vi "SWERVE_SIM_MODULE_READ_ENCODERS.vi"(10 "FPGA_Time_Seconds":dbl=-1.0, 11 "Swerve Module TypDef":T1) -> (2 "Swerve Distance_Radians":dbl, 3 "Wheel Distance_Meters":dbl)   [LabVIEW 2019]
uses:
  <vilib>/Rock Robotics/WPI/ThirdParty/JAS_Junk/TrajLib/Trajectory_Library.lvlib
  <vilib>/Rock Robotics/SystemInterfaces/Encoder/FPGA_EncoderIdx.ctl
  <vilib>/Rock Robotics/WPI/Encoder/WPI_EncoderType.ctl
  <vilib>/Rock Robotics/SystemInterfaces/Counter/FPGA_CounterCtrSystemIndex.ctl
  <vilib>/Rock Robotics/WPI/Encoder/WPI_EncoderDevRef.ctl
  <vilib>/Rock Robotics/SystemInterfaces/DIO/FPGA_DIOPWMChannel.ctl
  <vilib>/Rock Robotics/WPI/PWM/WPI_PWMDeadband.ctl
  <vilib>/Rock Robotics/WPI/MotorControl/WPI_MotorControlType.ctl
  <vilib>/Rock Robotics/SystemInterfaces/DIO/FPGA_DIOChannel.ctl
  <vilib>/Rock Robotics/WPI/MotorControl/WPI_MotorControlDeviceRef.ctl
  Swerve_Drive_System/SWERVE_DRIVE_MODULE_TYPDEF.ctl
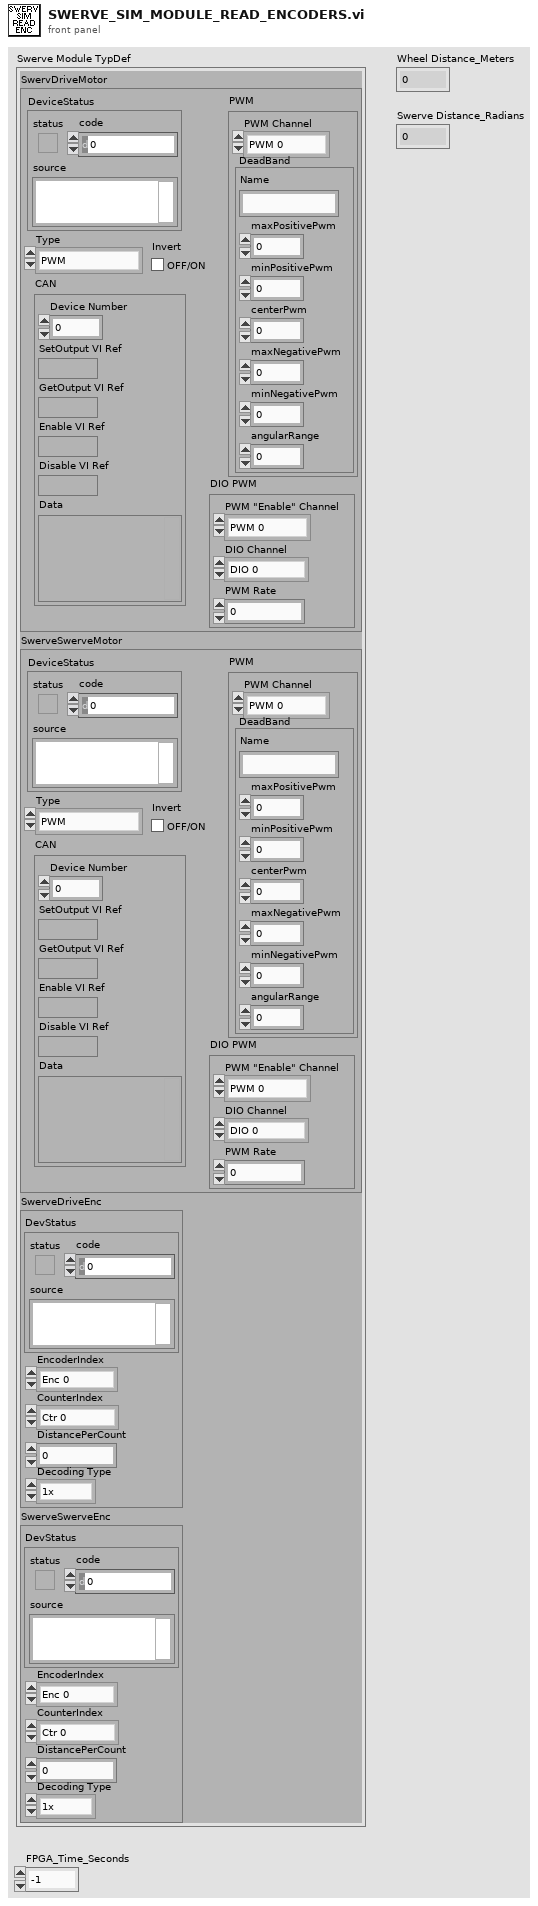
[diagram p1: front panel]
types:
  T1 = typedef "SWERVE_DRIVE_MODULE_TYPDEF.ctl" = cluster{"SwervDriveMotor":T2, "SwerveSwerveMotor":T2, "SwerveDriveEnc":T7, "SwerveSwerveEnc":T7}
  T2 = typedef "WPI_MotorControlDeviceRef.ctl" = cluster{"DeviceStatus":errorcluster, "Type":T3, "PWM":cluster{"PWM Channel":T4, "DeadBand":T5}, "CAN":cluster{"Device Number":u8, "SetOutput VI Ref":variant, "GetOutput VI Ref":variant, "Enable VI Ref":variant, "Disable VI Ref":variant, "Data":variant}, "Invert":bool, "DIO PWM":cluster{"PWM \"Enable\" Channel":T4, "DIOChannel":T6, "PWM Rate":dbl}}
  T3 = typedef "WPI_MotorControlType.ctl" = enum16{"PWM", "CAN", "DIO PWM"}
  T4 = typedef "FPGA_DIOPWMChannel.ctl" = enum8{"PWM 0", "PWM 1", "PWM 2", "PWM 3", "PWM 4", "PWM 5", "PWM 6", "PWM 7", "PWM 8", "PWM 9", "PWM MXP 0", "PWM MXP 1", "PWM MXP 2", "PWM MXP 3", "PWM MXP 4", "PWM MXP 5", "PWM MXP 6", "PWM MXP 7", "PWM MXP 8", "PWM MXP 9", "Invalid"}
  T5 = typedef "WPI_PWMDeadband.ctl" = cluster{"Name":string, "maxPositivePwm":i32, "minPositivePwm":i32, "centerPwm":i32, "maxNegativePwm":i32, "minNegativePwm":i32, "angularRange":u16}
  T6 = typedef "FPGA_DIOChannel.ctl" = enum8{"DIO 0", "DIO 1", "DIO 2", "DIO 3", "DIO 4", "DIO 5", "DIO 6", "DIO 7", "DIO 8", "DIO 9", "DIO MXP 0", "DIO MXP 1", "DIO MXP 2", "DIO MXP 3", "DIO MXP 4", "DIO MXP 5", "DIO MXP 6", "DIO MXP 7", "DIO MXP 8", "DIO MXP 9", "DIO MXP 10", "DIO MXP 11", "DIO MXP 12", "DIO MXP 13", "DIO MXP 14", "DIO MXP 15", "SPI Port CS1", "SPI Port CS2", "SPI Port CS3", "SPI Port MISO", "SPI Port MOSI", "Invalid"}
  T7 = typedef "WPI_EncoderDevRef.ctl" = cluster{"DevStatus":errorcluster, "EncoderIndex":T8, "CounterIndex":T9, "DistancePerCount":dbl, "Decoding Type":T10}
  T8 = typedef "FPGA_EncoderIdx.ctl" = enum8{"Enc 0", "Enc 1", "Enc 2", "Enc 3", "Enc 4", "Enc 5", "Enc 6", "Enc 7", "Invalid"}
  T9 = typedef "FPGA_CounterCtrSystemIndex.ctl" = enum8{"Ctr 0", "Ctr 1", "Ctr 2", "Ctr 3", "Ctr 4", "Ctr 5", "Ctr 6", "Ctr 7", "Invalid"}
  T10 = typedef "WPI_EncoderType.ctl" = enum16{"1x", "2x", "4x"}
  T11 = typedef "SWERVE_SIM_MODULE_MOTOR_CO.ctl" = cluster{"WheelMotorDmd":dbl, "SwerveMotorDmd":dbl}
  T12 = typedef "SWERVE_SIM_MODULE_MOTOR_PV.ctl" = cluster{"WheelMotorSpd":dbl, "SwerveMotorSpd":dbl, "WheelDist":dbl, "SwerveAngle":dbl}
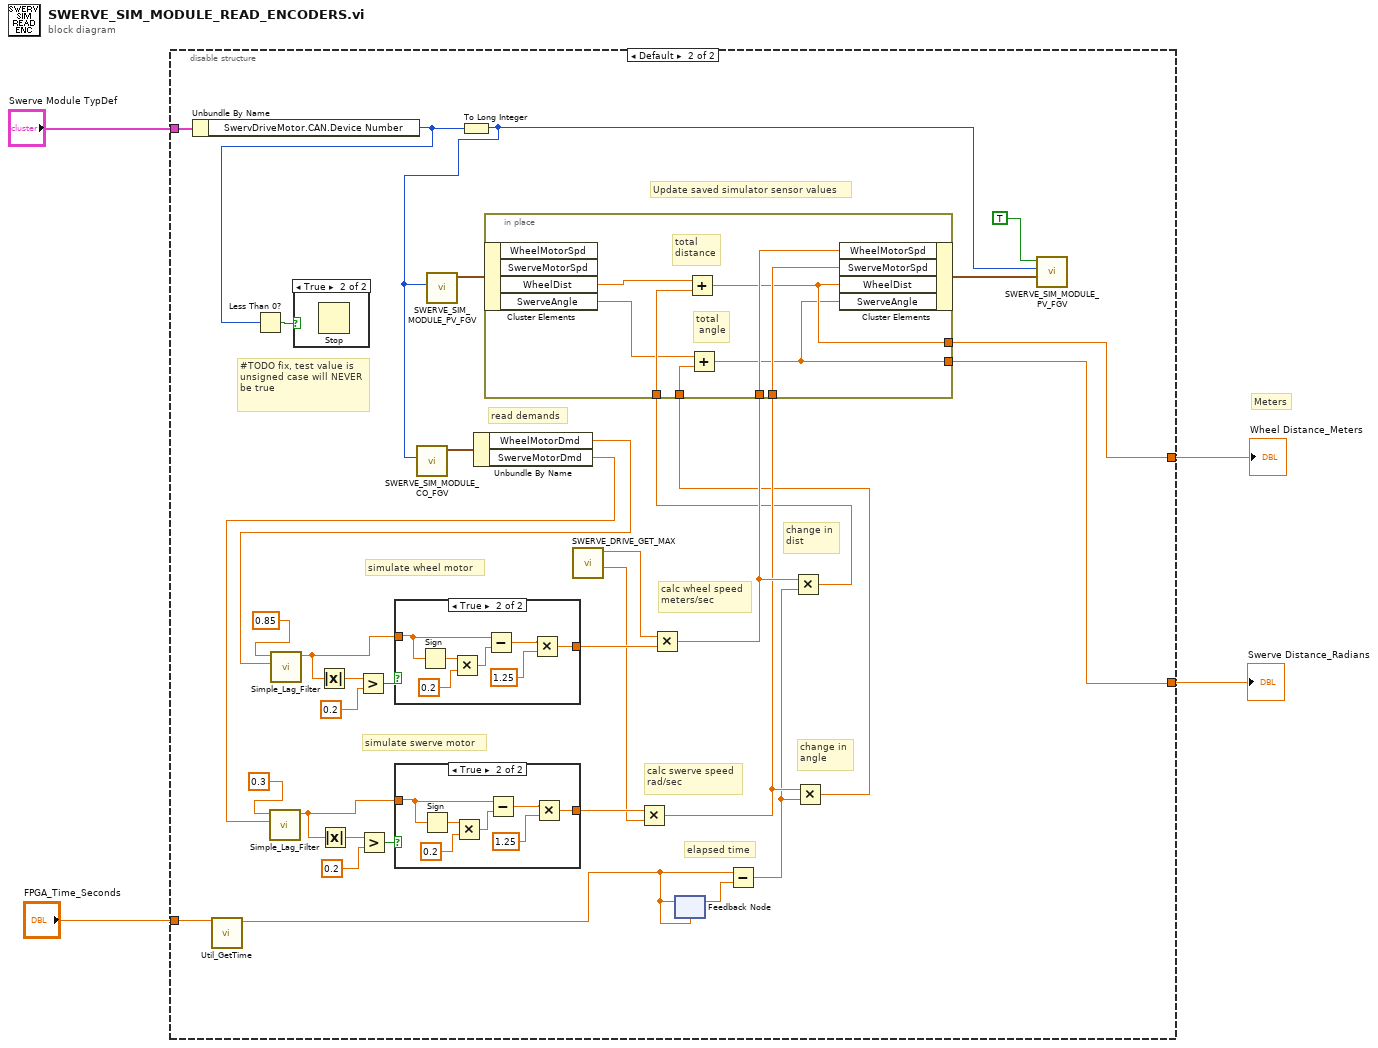
[diagram p0: block diagram]
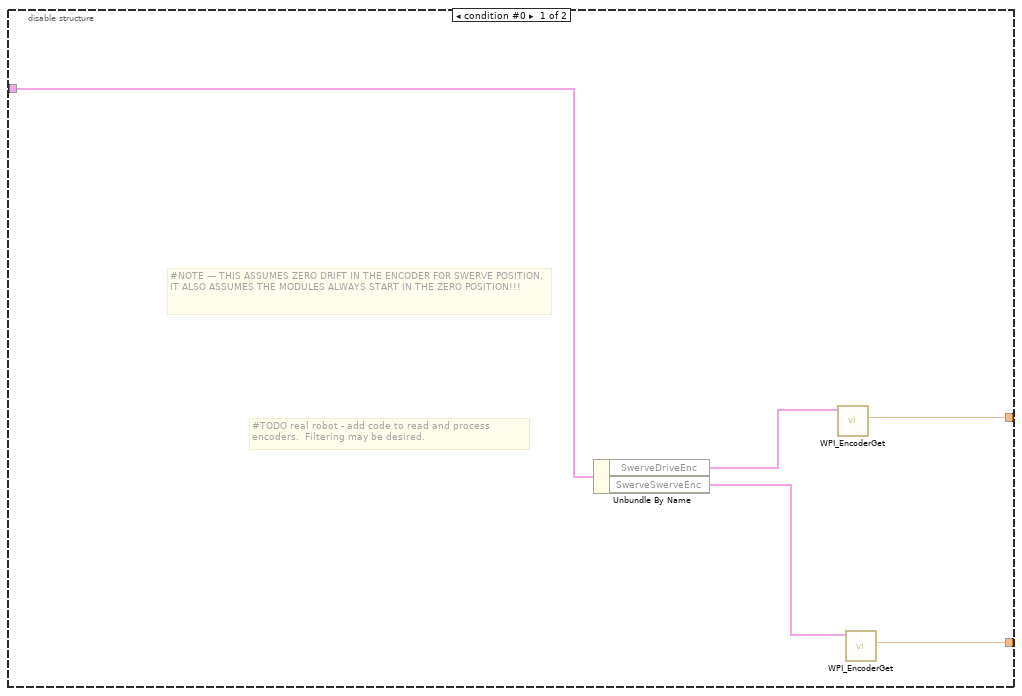
[diagram p2: hidden frame]
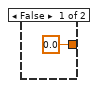
[diagram p3: hidden frame]
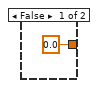
[diagram p4: hidden frame]
diagram:
  # "Meters"
  n1 = disable-structure shown="Default" {
    disable-tunnel: [w7 w11] -> w3
    disable-tunnel: [w6 w10] -> w2
    disable-tunnel: "Swerve Module TypDef" -> [w5 w43]
    disable-tunnel: "FPGA_Time_Seconds" -> [_ w17]
    frame condition #0 {
      # "#TODO real robot - add code to read and process encoders.  Filtering may be desired."
      # "#NOTE --- THIS ASSUMES ZERO DRIFT IN THE ENCODER FOR SWERVE POSITION.  IT ALSO ASSUMES THE MODULES ALWAYS START IN THE ZERO POSITION!!!"
      n2 = Unbundle By Name(w5) -> ("SwerveDriveEnc"=w8:T7, "SwerveSwerveEnc"=w9:T7)
      n3 = call <vilib>:"WPI_EncoderGet.vi"("EncoderDevRef"=w8) -> ("Distance"=w7:dbl)  [unwired: 5 in, 5 out]
      n4 = call <vilib>:"WPI_EncoderGet.vi"("EncoderDevRef"=w9) -> ("Distance"=w6:dbl)  [unwired: 5 in, 5 out]
    }
    frame condition #1 (active) {
      # "Update saved simulator sensor values"
      # "change in\nangle"
      # "change in\ndist"
      # "calc wheel speed\nmeters/sec"
      # "calc swerve speed\nrad/sec"
      # "simulate swerve motor"
      # "simulate wheel motor"
      # "#TODO fix, test value is unsigned case will NEVER be true"
      # "elapsed time"
      # "read demands"
      n5 = Unbundle By Name(w43) -> ("SwervDriveMotor.CAN.Device Number"=w21:u8)
      n6 = call <vilib>:"Util_GetTime.vi"("Pass_Through_Time"=w17) -> ("FPGA_Time_Seconds"=w16:dbl)  [unwired: 9 in, 1 out]
      n7 = Less Than 0?(x=w21) -> (x < 0?=w38:bool)
      n8 = case shown="True" w38 {
        frame False {
        }
        frame True {
          n9 = Stop() -> ()  [unwired: 1 in]
        }
      }
      n10 = To Long Integer(number=w21) -> (32bit integer=w20:i32)
      n11 = call "SWERVE_SIM_MODULE_CO_FGV.vi"("Index"=w20) -> ("out SwerveModuleMotorDmd"=w39:T11)  [unwired: 10 in]
      n12 = call "SWERVE_SIM_MODULE_PV_FGV.vi"("Index"=w20) -> ("Out SwerveModulePV"=w15:T12)  [unwired: 10 in]
      n13 = Unbundle By Name(w39) -> ("WheelMotorDmd"=w27:dbl, "SwerveMotorDmd"=w34:dbl)
      n14 = call "Simple_Lag_Filter.vi"("Input"=w34, "Lag"=0.3) -> ("Lagged Ouptut"=w33:dbl)  [unwired: 9 in]
      n15 = call "Simple_Lag_Filter.vi"("Input"=w27, "Lag"=0.85) -> ("Lagged Ouptut"=w28:dbl)  [unwired: 9 in]
      n16 = Absolute Value(x=w28) -> (abs(x)=w31:dbl)
      n17 = Absolute Value(x=w33) -> (abs(x)=w37:dbl)
      n18 = Greater?(x=w31, y=0.2) -> (0:w29:bool)
      n19 = Greater?(x=w37, y=0.2) -> (0:w35:bool)
      n20 = case shown="True" w29 {
        tunnel: w28 -> [_ w57]
        tunnel: [0.0 w53] -> w26
        frame False {
        }
        frame True {
          n21 = Sign(1:w57) -> (0:w59:dbl)
          n22 = Multiply(x=w59, y=0.2) -> (x*y=w56:dbl)
          n23 = Subtract(x=w57, y=w56) -> (x-y=w55:dbl)
          n24 = Multiply(x=w55, y=1.25) -> (x*y=w53:dbl)
        }
      }
      n25 = case shown="True" w35 {
        tunnel: w33 -> [_ w65]
        tunnel: [0.0 w61] -> w32
        frame False {
        }
        frame True {
          n26 = Sign(1:w65) -> (0:w67:dbl)
          n27 = Multiply(x=w67, y=0.2) -> (x*y=w64:dbl)
          n28 = Subtract(x=w65, y=w64) -> (x-y=w63:dbl)
          n29 = Multiply(x=w63, y=1.25) -> (x*y=w61:dbl)
        }
      }
      n30 = call "SWERVE_DRIVE_GET_MAX.vi"() -> ("Max Rotational Vel (Rad/Sec)"=w22:dbl, "Max Wheel Vel (Meter/Sec)"=w25:dbl)  [unwired: 10 in]
      n31 = Multiply(x=w32, y=w22) -> (x*y=w40:dbl)
      n32 = Multiply(x=w25, y=w26) -> (x*y=w41:dbl)
      n33 = feedback #1(w16) -> (w24:dbl)
      n34 = feedback-in #1(w16) -> ()
      n35 = Subtract(x=w16, y=w24) -> (x-y=w23:dbl)
      n36 = Multiply(x=w41, y=w23) -> (x*y=w13:dbl)
      n37 = Multiply(x=w40, y=w23) -> (x*y=w12:dbl)
      n38 = in-place {
        in-place-border: w41 -> [w51]
        in-place-border: w40 -> [w50]
        in-place-border: w13 -> [w48]
        in-place-border: w12 -> [w46]
        in-place-border: [w45] -> w11
        in-place-border: [w44] -> w10
        # "total \ndistance"
        # "total\n angle"
        n39 = in-place-cluster #2(w15) -> ("WheelDist"=w49:dbl, "SwerveAngle"=w47:dbl)  [unwired: 2 out]
        n40 = Add(x=w49, y=w48) -> (x+y=w45:dbl)
        n41 = Add(x=w47, y=w46) -> (x+y=w44:dbl)
        n42 = in-place-cluster #2("WheelMotorSpd"=w51, "SwerveMotorSpd"=w50, "WheelDist"=w45, "SwerveAngle"=w44) -> (w14:T12)
      }
      n43 = call "SWERVE_SIM_MODULE_PV_FGV.vi"("In SwerveModulePV"=w14, "Index"=w20, "WRITE"=TRUE) -> ()  [unwired: 8 in, 1 out]
    }
  }
  "Wheel Distance_Meters" <- w3
  "Swerve Distance_Radians" <- w2
